vi "LJUD UE9RAW ReadMem.vi"(7 "Comm Settings":T1={"Open LabJack "=TRUE, "Use USB"=TRUE, "IP Address"="192.168.1.209", "PortA"=52360, "PortB"=0}, 8 "error in (no error)":errorcluster, 10 "BlockNum":u8, 11 "Handle In":i32) -> (0 "error out":errorcluster, 1 "Mem Data":u8[](array[numeric]), 3 "Handle Out":i32)   [LabVIEW 2021]
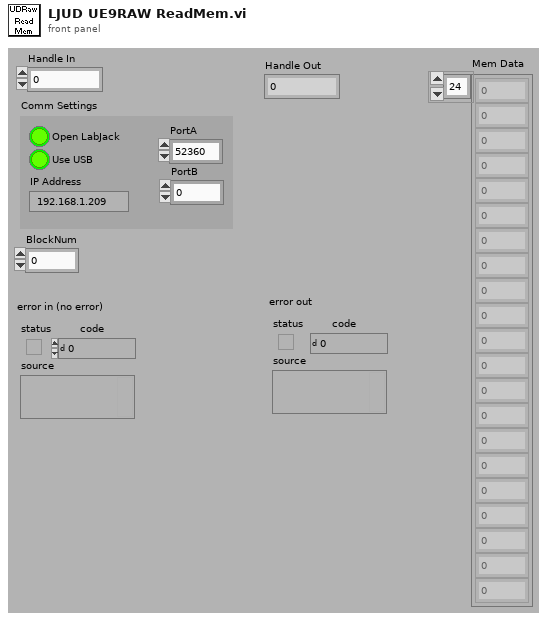
[diagram p1: front panel]
types:
  T1 = cluster{"Open LabJack ":bool, "Use USB":bool, "IP Address":string, "PortA":u16, "PortB":u16}
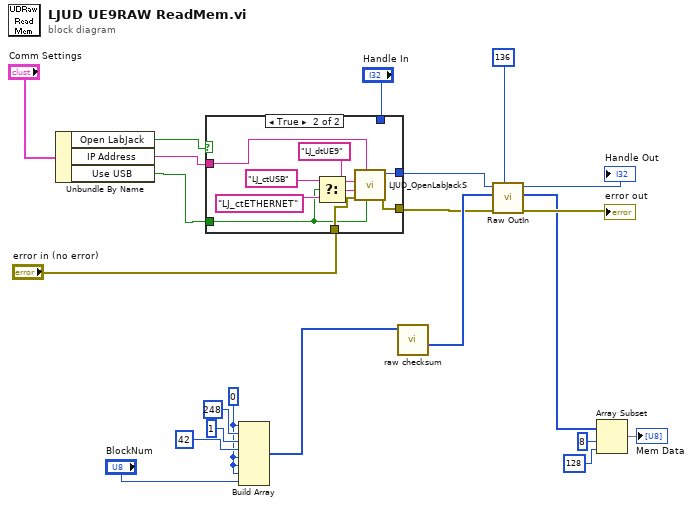
[diagram p0: block diagram]
diagram:
  w17 = u8 0 ("Input Element")
  n1 = Unbundle By Name("Comm Settings") -> ("Open LabJack"=w1:bool, "IP Address"=w2:string, "Use USB"=w3:bool)
  n2 = case shown="True" w1 {
    tunnel: w2 -> [_ w27]
    tunnel: "error in (no error)" -> [w24 w31]
    tunnel: [w24 w30] -> w6
    tunnel: [w23 w28] -> w7
    tunnel: w3 -> [_ w29]
    tunnel: "Handle In" -> [w23 _]
    frame False {
    }
    frame True {
      n3 = Select(t="LJ_ctUSB" ("ConnectionType"), s=w29, f="LJ_ctETHERNET" ("ConnectionType")) -> (s? t:f=w25:string)
      n4 = call "LJUD_OpenLabJackS.vi"("FirstFound"=w29, "Address"=w27, "error in"=w31, "ConnectionType"=w25, "DeviceType"="LJ_dtUE9") -> ("error out"=w30:errorcluster, "Handle"=w28:i32)  [unwired: 4 in, 1 out]
    }
  }
  n5 = Build Array(w17, u8 248 ("Input Element"), u8 1 ("Input Element"), u8 42 ("Input Element"), w17, w17, w17, "BlockNum") -> (w19:u8[])
  n6 = call "raw checksum.vi"("Array"=w19) -> ("Array Output"=w9:u8[])  [unwired: 3 in, 7 out]
  n7 = call "Raw OutIn.vi"("# of bytes to read in"=136 ("# of bytes to read"), "error in"=w6, "Raw Out"=w9, "Handle In"=w7) -> ("error out"=→"error out":errorcluster, "Raw In"=w10:u8[], "Handle Out"=→"Handle Out":i32)  [unwired: 4 in, 1 out]
  n8 = Array Subset(array=w10, index=8 ("Array Index"), length=128 ("Array Length")) -> (→"Mem Data":u8[])
